vi "InitializeMaskLoad.vi"(4 "dxfFile":string, 5 "Masks":string, 6 "WaferTestPoints":string, 7 "DXFCanvas":refnum<k24>, 9 "TestPointsLoaded":bool, 10 "Wafer Definition File":path, 11 "MicrositesRef":refnum<k24>) -> (0 "error out":errorcluster, 3 "error out 5":errorcluster)   [LabVIEW 2020]
uses:
  C:/Projects/RaxTagServer/LabviewDXFViewer/LabviewDXFViewer/bin/Release/LabviewDXFViewer.exe
  LabviewDXFViewer/bin/Release/LabviewDXFViewer.exe
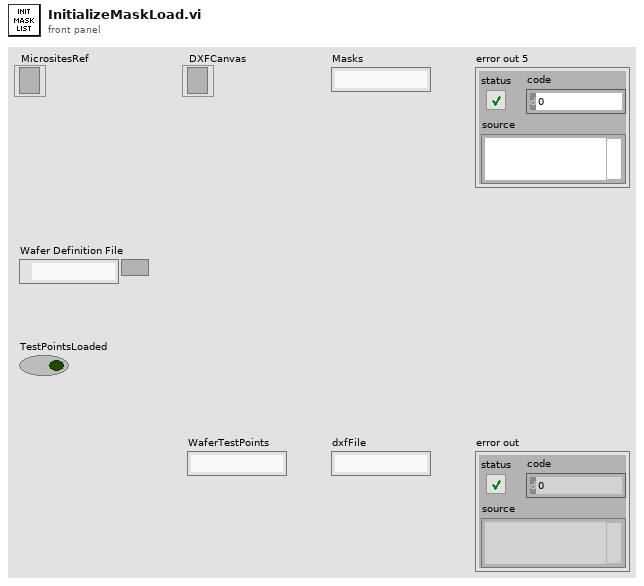
[diagram p1: front panel]
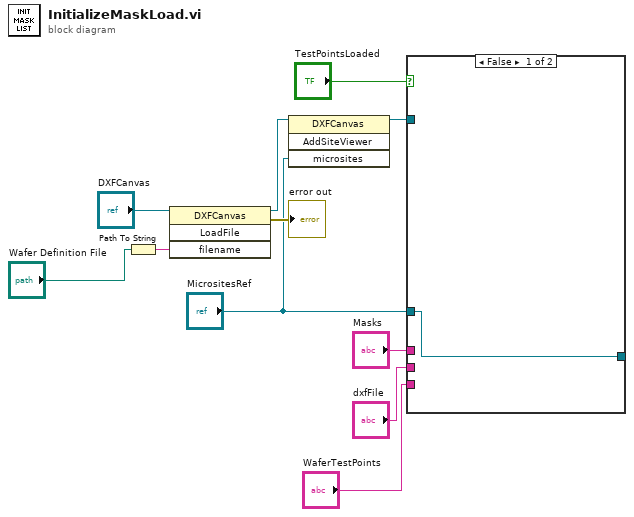
[diagram p0: block diagram]
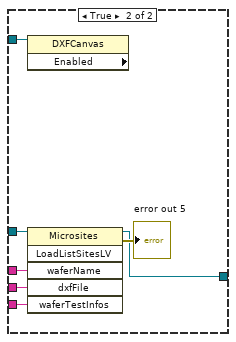
[diagram p2: hidden frame]
diagram:
  n1 = Path To String(path="Wafer Definition File") -> (string=w4:string)
  n2 = invoke class="DXFCanvas" method="LoadFile"(reference="DXFCanvas", "filename"=w4) -> (reference out=w2:refnum<k24>, error out=→"error out":errorcluster)  [unwired: 2 in, 2 out]
  n3 = invoke class="DXFCanvas" method="AddSiteViewer"(reference=w2, "microsites"="MicrositesRef") -> (reference out=w9:refnum<k24>)  [unwired: 2 in, 3 out]
  n4 = case shown="False" "TestPointsLoaded" {
    tunnel: "Masks" -> [_ w19]
    tunnel: "MicrositesRef" -> [w12 w18]
    tunnel: w9 -> [_ w16]
    tunnel: "WaferTestPoints" -> [_ w15]
    tunnel: "dxfFile" -> [_ w14]
    tunnel: [w12 w13] -> _
    frame False {
    }
    frame True {
      n5 = property class="DXFCanvas" props=["Enabled"](reference=w16) -> ()  [unwired: 1 in, 3 out]
      n6 = invoke class="Microsites" method="LoadListSitesLV"(reference=w18, "waferName"=w19, "dxfFile"=w14, "waferTestInfos"=w15) -> (reference out=w13:refnum<k24>, error out=→"error out 5":errorcluster)  [unwired: 2 in, 4 out]
    }
  }
